vi "CreateEventsForStatus.vi"() -> (2 "Event Registration Refnum":refnum<event-registration>, 3 "Events":T1)   [LabVIEW 2020, in "SolutionBuilder.lvlib"]
uses:
  SolutionBuilder/SolutionBuilder.lvlib
  SolutionBuilder/Events.ctl
  SolutionBuilder/EventUpdateList.ctl
  SolutionBuilder/EventItemBuilt.ctl
  SolutionBuilder/SolutionBuilder.lvclass
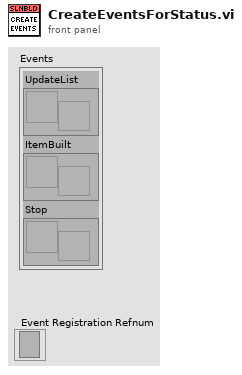
[diagram p1: front panel]
types:
  T1 = typedef "SolutionBuilder.lvlib/Events.ctl" = cluster{"UpdateList":T2, "ItemBuilt":T3, "Stop":refnum<user-event>}
  T2 = typedef "SolutionBuilder.lvlib/SolutionBuilder.lvclass/EventUpdateList.ctl" = refnum<user-event>
  T3 = typedef "SolutionBuilder.lvlib/SolutionBuilder.lvclass/EventItemBuilt.ctl" = refnum<user-event>
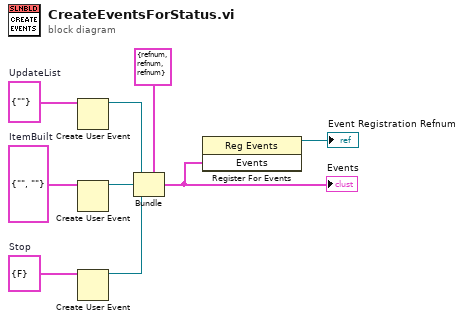
[diagram p0: block diagram]
diagram:
  w7 = cluster{"Item":string} {"Item"=""}  # UpdateList
  w6 = cluster{"Stop":bool} {"Stop"=FALSE}  # Stop
  w5 = cluster{"Item":string, "Result":string} {"Item"="", "Result"=""}  # ItemBuilt
  n1 = Create User Event(user event datatype=w7) -> (user event=w8:refnum<user-event>)  [unwired: 1 in, 1 out]
  n2 = Create User Event(user event datatype=w5) -> (user event=w9:refnum<user-event>)  [unwired: 1 in, 1 out]
  n3 = Create User Event(user event datatype=w6) -> (user event=w4:refnum<user-event>)  [unwired: 1 in, 1 out]
  n4 = Bundle(cluster=T1 {"UpdateList"=refnum, "ItemBuilt"=refnum, "Stop"=refnum} ("Events"), "UpdateList"=w8, "ItemBuilt"=w9, "Stop"=w4) -> (w2:T1)
  "Events" <- w2
  n5 = register-events(w2) -> (reference out=→"Event Registration Refnum":refnum<event-registration>)  [unwired: 2 in, 1 out]
